vi "USB5GetDi.vi"(8 "错误输入（无错误）":errorcluster, 9 "TimeOut":i32=2000, 10 "Points":u32, 11 "DevIndex":i32) -> (0 "错误输出":errorcluster, 1 "Di":u8[](array[numeric]) format="%04b", 2 "DiFifoUsed":i32, 3 "DevIndex Out":i32)   [LabVIEW 2020]
uses:
  USB5000.dll
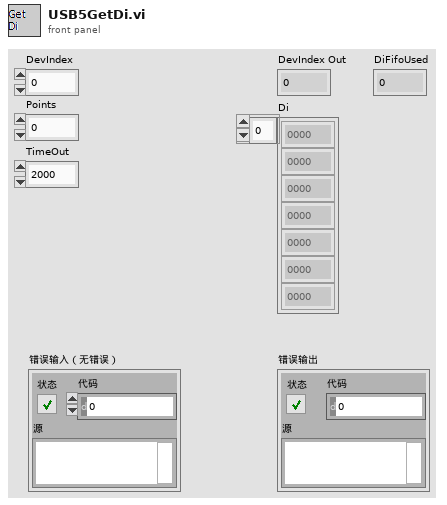
[diagram p1: front panel]
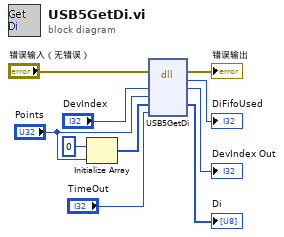
[diagram p0: block diagram]
diagram:
  n1 = Initialize Array(u8 0, "Points") -> (w3:u8[])
  n2 = dll-call lib="USB5000.dll" fn="USB5GetDi"(error in="错误输入（无错误）", "DevIndex"="DevIndex", "Points"="Points", "Di"=w3, "TimeOut"="TimeOut") -> (error out=→"错误输出":errorcluster, "返回类型"=→"DiFifoUsed":i32, "DevIndex"=→"DevIndex Out":i32, "Di"=→"Di":u8[])  [unwired: 4 in, 1 out]
